vi "Ramp Rate Coercion.vi"(9 "Requested Value":sgl, 10 "Original Value":sgl, 11 "Ramp Rate (W)":sgl) -> (3 "Coerced Value":sgl)   [LabVIEW 2018]
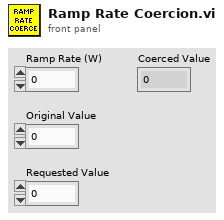
[diagram p1: front panel]
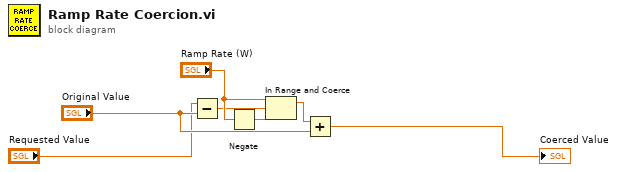
[diagram p0: block diagram]
diagram:
  n1 = Subtract(x="Requested Value", y="Original Value") -> (x-y=w2:sgl)
  n2 = Negate(x="Ramp Rate (W)") -> (-x=w4:sgl)
  n3 = In Range and Coerce(upper limit="Ramp Rate (W)", x=w2, lower limit=w4) -> (coerced(x)=w5:sgl)  [unwired: 1 out]
  n4 = Add(x=w5, y="Original Value") -> (x+y=→"Coerced Value":sgl)
